vi "Set_Sequence_Argument.vi"(2 "Enable":bool, 3 "Argument":string, 4 "Index":i32, 5 "Input Sequence":cluster{string, string[], dbl[], dbl}[](array[cluster])) -> (0 "Argument String":string, 1 "Output Sequence":cluster{string, string[], dbl[], dbl}[](array[cluster]))   [LabVIEW 2011]
doc: "This VI sets a boolean argument in the context of an entire sequence. It is identical to Set_Argument.vi, but instead of operating on an event directly, it operates on an element in the sequence determined by the \"Index\" parameter."
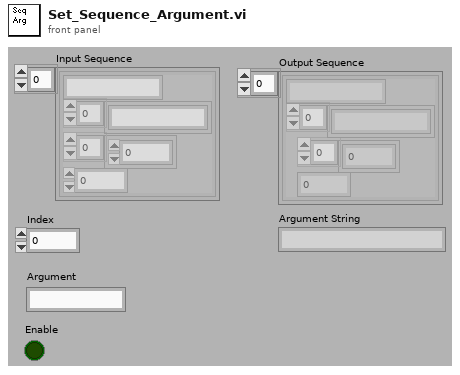
[diagram p1: front panel]
types:
  T1 = cluster{string, "Argument List Out":string[], dbl[], dbl}
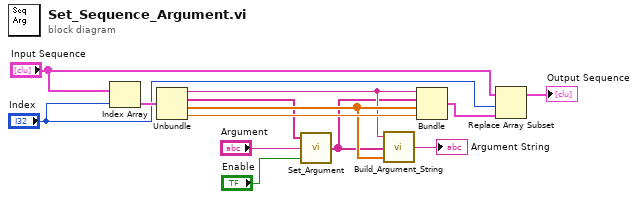
[diagram p0: block diagram]
diagram:
  n1 = Index Array(array="Input Sequence", index="Index") -> (element=w13:cluster{string, string[], dbl[], dbl})
  n2 = Unbundle(w13) -> (w5:string, w4:string[], w6:dbl[], w12:dbl)
  n3 = call "Set_Argument.vi"("Enable"="Enable", "Argument"="Argument", "Argument List In"=w4) -> ("Argument List Out"=w3:string[])
  n4 = call "Build_Argument_String.vi"("Flow Array"=w6, "Argument List"=w3, "Command"=w5) -> ("Argument String"=→"Argument String":string)
  n5 = Bundle(w5, "Argument List Out"=w3, w6, w12) -> (w11:T1)  [unwired: 1 out]
  n6 = Replace Array Subset(array="Input Sequence", new element=w11, index="Index") -> (→"Output Sequence":cluster{string, string[], dbl[], dbl}[])
